vi "Test Demonstration of Configuration file Sequential Read.vi"(8 "error in (no error)":errorcluster, 11 "Configuration File Process Interface Test In":refnum<class "Configuration File Process Interface Test.lvclass">) -> (0 "error out":errorcluster, 3 "Configuration File Process Interface Test Out":refnum<class "Configuration File Process Interface Test.lvclass">)   [LabVIEW 2020]
uses:
  7a9225b6-cacd-4ceb-ab20-9a24fc8ee0db.vi
  Mock Configurable Process/Mock Configurable Process.lvclass
  Configuration File Process Interface Test.lvclass
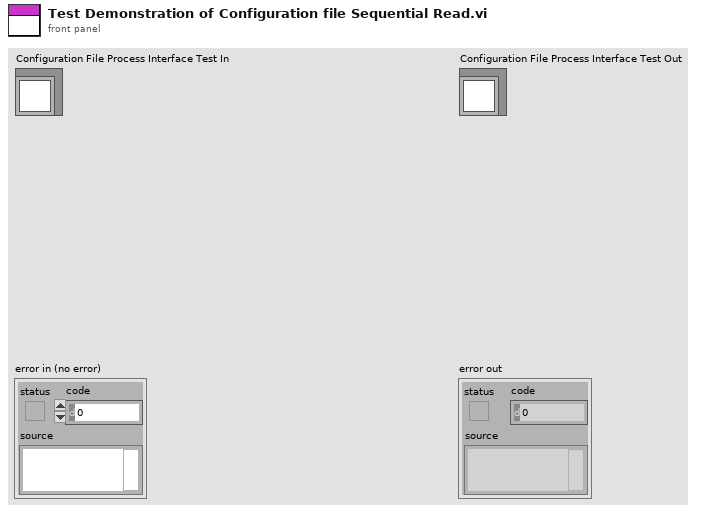
[diagram p1: front panel]
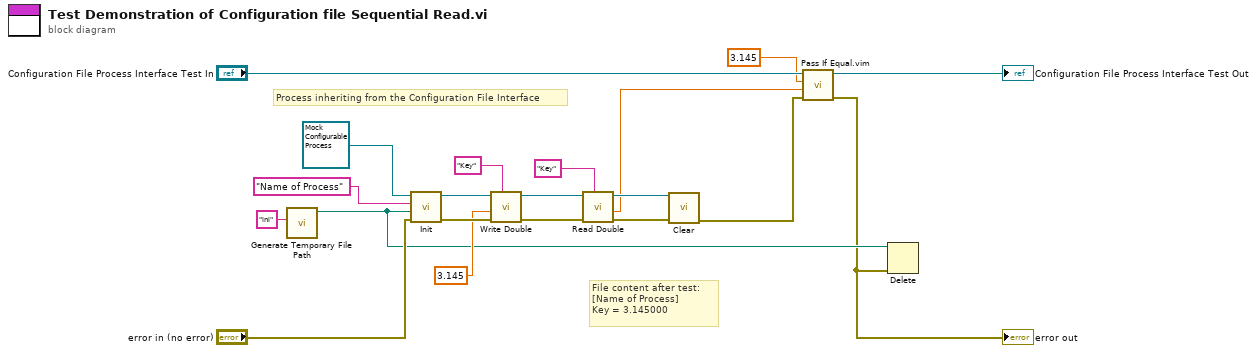
[diagram p0: block diagram]
diagram:
  # "File content after test:\n[Name of Process]\nKey = 3.145000"
  # "Process inheriting from the Configuration File Interface"
  n1 = call <vilib>:"Generate Temporary File Path.vi"("Temporary File Extension (tmp)"="ini") -> ("Unique Temporary File Path"=w2:path)  [unwired: 9 in, 1 out]
  n2 = call-dynamic "Init.vi"("error in (no error)"="error in (no error)", "Config File Path"=w2, "Name"="Name of Process", "Process In"=refnum<class "Mock Configurable Process.lvclass"> refnum ("Mock Configurable.lvclass")) -> ("error out"=w16:errorcluster, "Process Out"=w15:refnum<class "Mock Configurable Process.lvclass">)  [unwired: 6 in]
  n3 = call-dynamic "Write Double.vi"("key"="Key", "error in (no error)"=w16, "Value"=3.145, "Configuration File In"=w15) -> ("error out"=w10:errorcluster, "Configuration File Out"=w11:refnum<class "Mock Configurable Process.lvclass">)  [unwired: 6 in]
  n4 = call-dynamic "Read Double.vi"("key"="Key", "error in (no error)"=w10, "Configuration File In"=w11) -> ("error out"=w9:errorcluster, "value"=w4:dbl, "Configuration File Out"=w8:refnum<class "Mock Configurable Process.lvclass">)  [unwired: 6 in]
  n5 = call-dynamic "Clear.vi"("error in (no error)"=w9, "Process In"=w8) -> ("error out"=w6:errorcluster)  [unwired: 9 in]
  n6 = call "Pass If Equal.vim"("error in (no error)"=w6, "Actual"=w4, "Expected"=3.145 ("Value"), "LUnit Test Case In"="Configuration File Process Interface Test In") -> ("error out"=w1:errorcluster, "LUnit Test Case Out"=→"Configuration File Process Interface Test Out":refnum<class "Configuration File Process Interface Test.lvclass">)  [unwired: 6 in]
  "error out" <- w1
  n7 = Delete(path (use dialog)=w2, error in=w1) -> ()  [unwired: 3 in, 3 out]
